vi "Part 2.vi"(11 "Input":string) -> (3 "Output":i64)   [LabVIEW 2021]
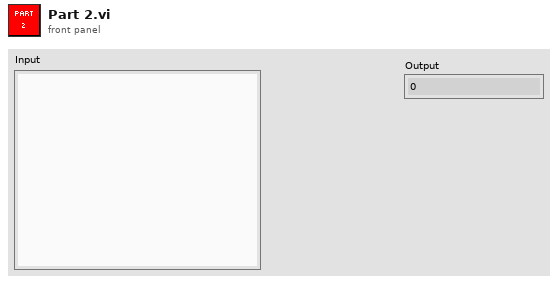
[diagram p1: front panel]
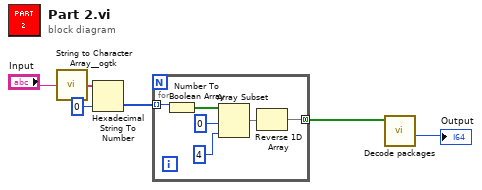
[diagram p0: block diagram]
diagram:
  n1 = call <userlib>:"String to Character Array__ogtk.vi"("Input String"="Input") -> ("Character Array"=w6:string[])
  n2 = Hexadecimal String To Number(string=w6, default (0uL)=u8 0 ("default (0 U32)")) -> (number=w4:u8[])  [unwired: 1 in, 1 out]
  n3 = for {
    tunnel: w4 -> [w12] mode=indexing
    tunnel: [w7] -> w3 mode=concatenating
    n4 = Number To Boolean Array(number=w12) -> (Boolean array=w11:bool[])
    n5 = Array Subset(array=w11, index=0, length=4) -> (w8:bool[])
    n6 = Reverse 1D Array(array=w8) -> (reversed array=w7:bool[])
  }
  n7 = call "Decode packages.vi"("Array"=w3) -> ("Value Out"=→"Output":u64)  [unwired: 8 in, 2 out]
